vi "Set Clip Size.vi"(8 "error in (no error)":errorcluster, 10 "Clip Size":cluster{"Hight":dbl, "Width":dbl}, 11 "Actor in":refnum<class "Actor.lvclass">) -> (0 "error out":errorcluster, 3 "Actor out":refnum<class "Actor.lvclass">)   [LabVIEW 2015, in "Actor.lvclass"]
uses:
  Actor.lvclass
  Actor.lvclass/Actor.ctl
  ImageOperaion/ImageOperation.lvclass/ImageOperation.ctl
  ImageOperaion/ImageOperation.lvclass
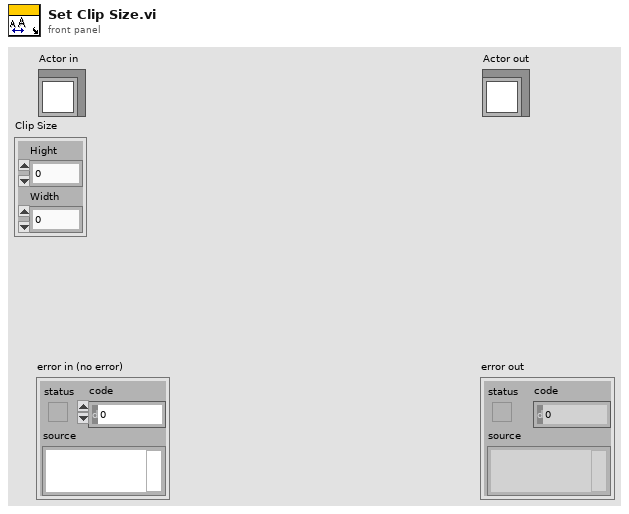
[diagram p1: front panel]
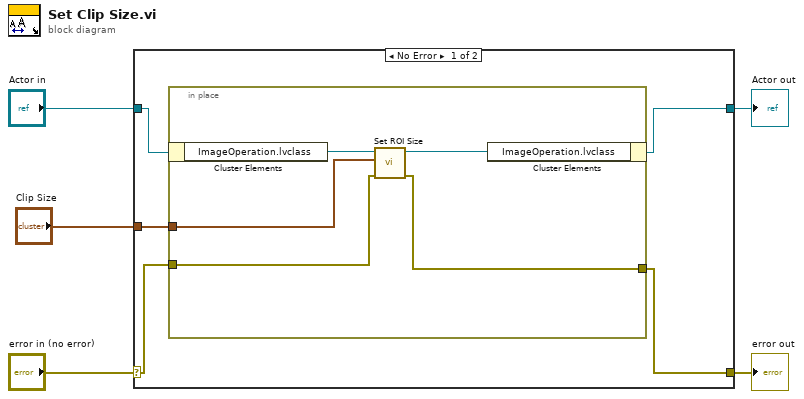
[diagram p0: block diagram]
diagram:
  n1 = case shown="No Error" "error in (no error)" {
    selector: "error in (no error)" -> [w8 w17]
    tunnel: [w7 w17] -> w4
    tunnel: [w6 w16] -> w2
    tunnel: "Actor in" -> [w10 w16]
    tunnel: "Clip Size" -> [w9 _]
    frame No Error {
      n2 = in-place {
        in-place-border: w9 -> [w14]
        in-place-border: w8 -> [w13]
        in-place-border: [w11] -> w7
        n3 = in-place-cluster #1(w10) -> ("ImageOperation.lvclass"=w15:refnum<class "ImageOperation.lvclass">)
        n4 = call "Set ROI Size.vi"("error in (no error)"=w13, "Size"=w14, "ImageOperation in"=w15) -> ("error out"=w11:errorcluster, "ImageOperation out"=w12:refnum<class "ImageOperation.lvclass">)  [unwired: 7 in]
        n5 = in-place-cluster #1("ImageOperation.lvclass"=w12) -> (w6:refnum<class "Actor.lvclass">)
      }
    }
    frame Error {
    }
  }
  "error out" <- w4
  "Actor out" <- w2
